vi "Order_Size_Control.vi"(8 "New Data":T1 {"ЦАП, градС" format="%.3g"; "Тнагр, градС" format="%.3g"; "Q, мл" format="%.3g"; "Рдм, МПа" format="%.3g"; "Рэфф, МПа" format="%.3g"; "dL, мм" format="%.4f"; "R, Ом" format="%.4f"; "Ргор, МПа" format="%.2f град.С"; "Рпл2, МПа" format="Р2 %#.2f МПа"}, 9 "Order Size":u32, 11 "Old Array":T1[](array[typedef]) {"ЦАП, градС" format="%.3g"; "Тнагр, градС" format="%.3g"; "Q, мл" format="%.3g"; "Рдм, МПа" format="%.3g"; "Рэфф, МПа" format="%.3g"; "dL, мм" format="%.4f"; "R, Ом" format="%.4f"; "Ргор, МПа" format="%.2f град.С"; "Рпл2, МПа" format="Р2 %#.2f МПа"}) -> (0 "New Data":T1 {"ЦАП, градС" format="%.3g"; "Тнагр, градС" format="%.3g"; "Q, мл" format="%.3g"; "Рдм, МПа" format="%.3g"; "Рэфф, МПа" format="%.3g"; "dL, мм" format="%.4f"; "R, Ом" format="%.4f"; "Ргор, МПа" format="%.2f град.С"; "Рпл2, МПа" format="Р2 %#.2f МПа"}, 3 "New Array":T1[](array[typedef]) {"ЦАП, градС" format="%.3g"; "Тнагр, градС" format="%.3g"; "Q, мл" format="%.3g"; "Рдм, МПа" format="%.3g"; "Рэфф, МПа" format="%.3g"; "dL, мм" format="%.4f"; "R, Ом" format="%.4f"; "Ргор, МПа" format="%.2f град.С"; "Рпл2, МПа" format="Р2 %#.2f МПа"})   [LabVIEW 2023, in "Graph_data_collector.lvlib"]
uses:
  Graph_data_collector.lvlib
  Data Control.ctl
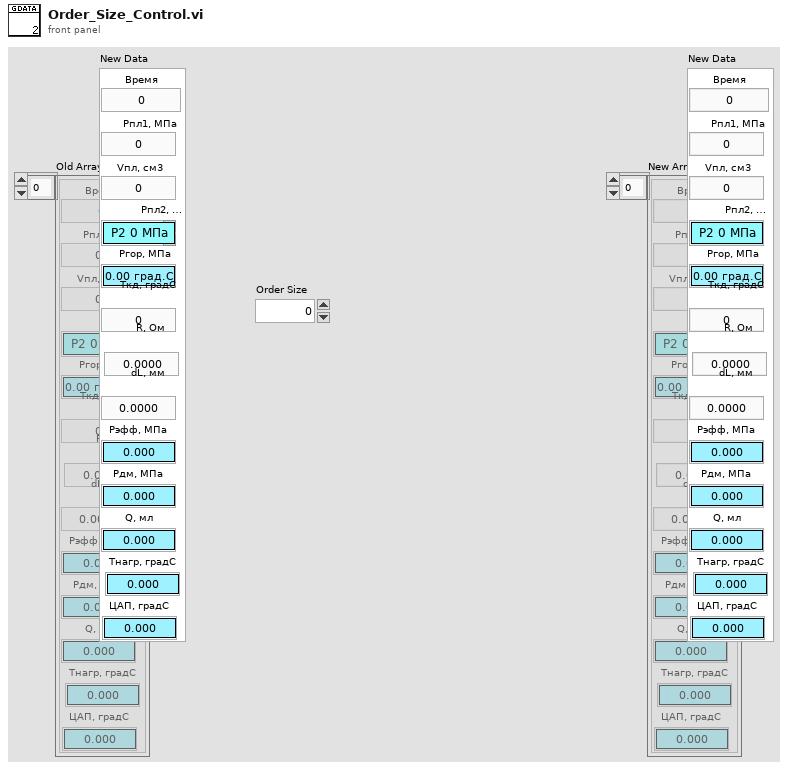
[diagram p1: front panel]
types:
  T1 = typedef "Graph_data_collector.lvlib/Data Control.ctl" = cluster{"Время":dbl, "Рпл1, МПа":dbl, "Vпл, см3":dbl, "Рпл2, МПа":dbl, "Ргор, МПа":dbl, "Ткд, градС":dbl, "R, Ом":dbl, "dL, мм":dbl, "Рэфф, МПа":dbl, "Рдм, МПа":dbl, "Q, мл":dbl, "Тнагр, градС":dbl, "ЦАП, градС":dbl}
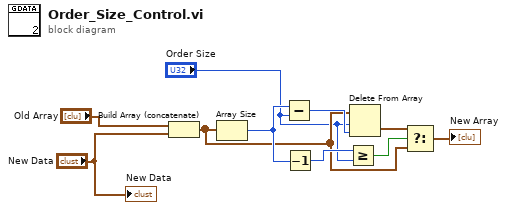
[diagram p0: block diagram]
diagram:
  n1 = Build Array (concatenate)("Old Array", "New Data") -> (w6:T1[])
  n2 = Array Size(array=w6) -> (size(s)=w8:i32)
  n3 = Subtract(x=w8, y="Order Size") -> (x-y=w10:u32)
  n4 = Decrement(x=w8) -> (x-1=w9:i32)
  n5 = Greater Or Equal?(x=w9, y="Order Size") -> (x >= y?=w5:bool)
  n6 = Delete From Array(array=w6, length="Order Size", index=w10) -> (deleted portion=w7:T1[])  [unwired: 1 out]
  n7 = Select(t=w7, s=w5, f=w6) -> (s? t:f=→"New Array":T1[])
  "New Data" <- "New Data"
